vi "CBSControlling.vi"() -> ()   [LabVIEW 2017]
uses:
  classes/DataHandlerMYiTOPS.lvclass
panel:
  out "Steps":u64
  out "NewVal":u64
  in  "Monitoring":T1 {"Meter" scale=0.0..20.0}
  out "appended array":string[](array[string])
  out "element":string
  out "Control-Matrix-Overview 2":i32(listbox)=-1
  in  "Controlling":T2={"LED 1"=FALSE, "Stop Client App"=FALSE, "LED 2"=FALSE, "Drive Motor"=FALSE, "Direcion Moter"=FALSE, "Steps"=512} {"Steps" min=1 step=1}
  in  "Cyber-physical Objects":i32(listbox)
  in  "Stop":bool
  out "Control-Matrix-Overview":i32(listbox)=-1
  # "Hard Key:"
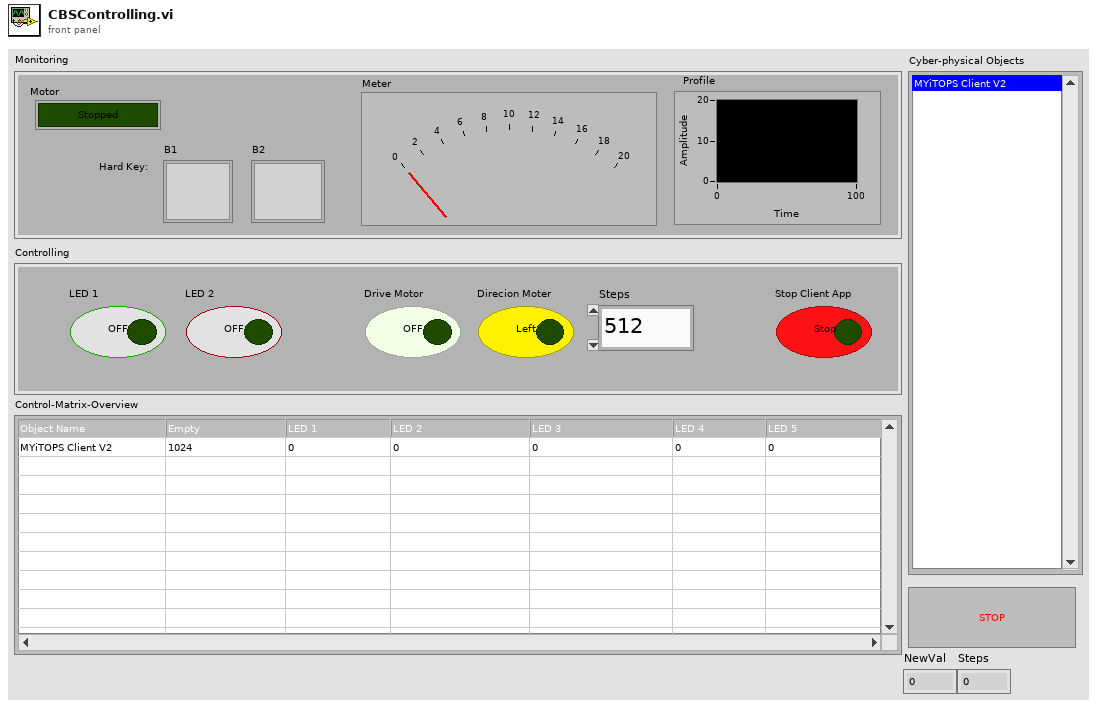
[diagram p1: front panel]
types:
  T1 = cluster{"Meter":i8, "Profile":dbl, "B2":bool, "B1":bool, "Motor":bool}
  T2 = cluster{"LED 1":bool, "Stop Client App":bool, "LED 2":bool, "Drive Motor":bool, "Direcion Moter":bool, "Steps":u64}
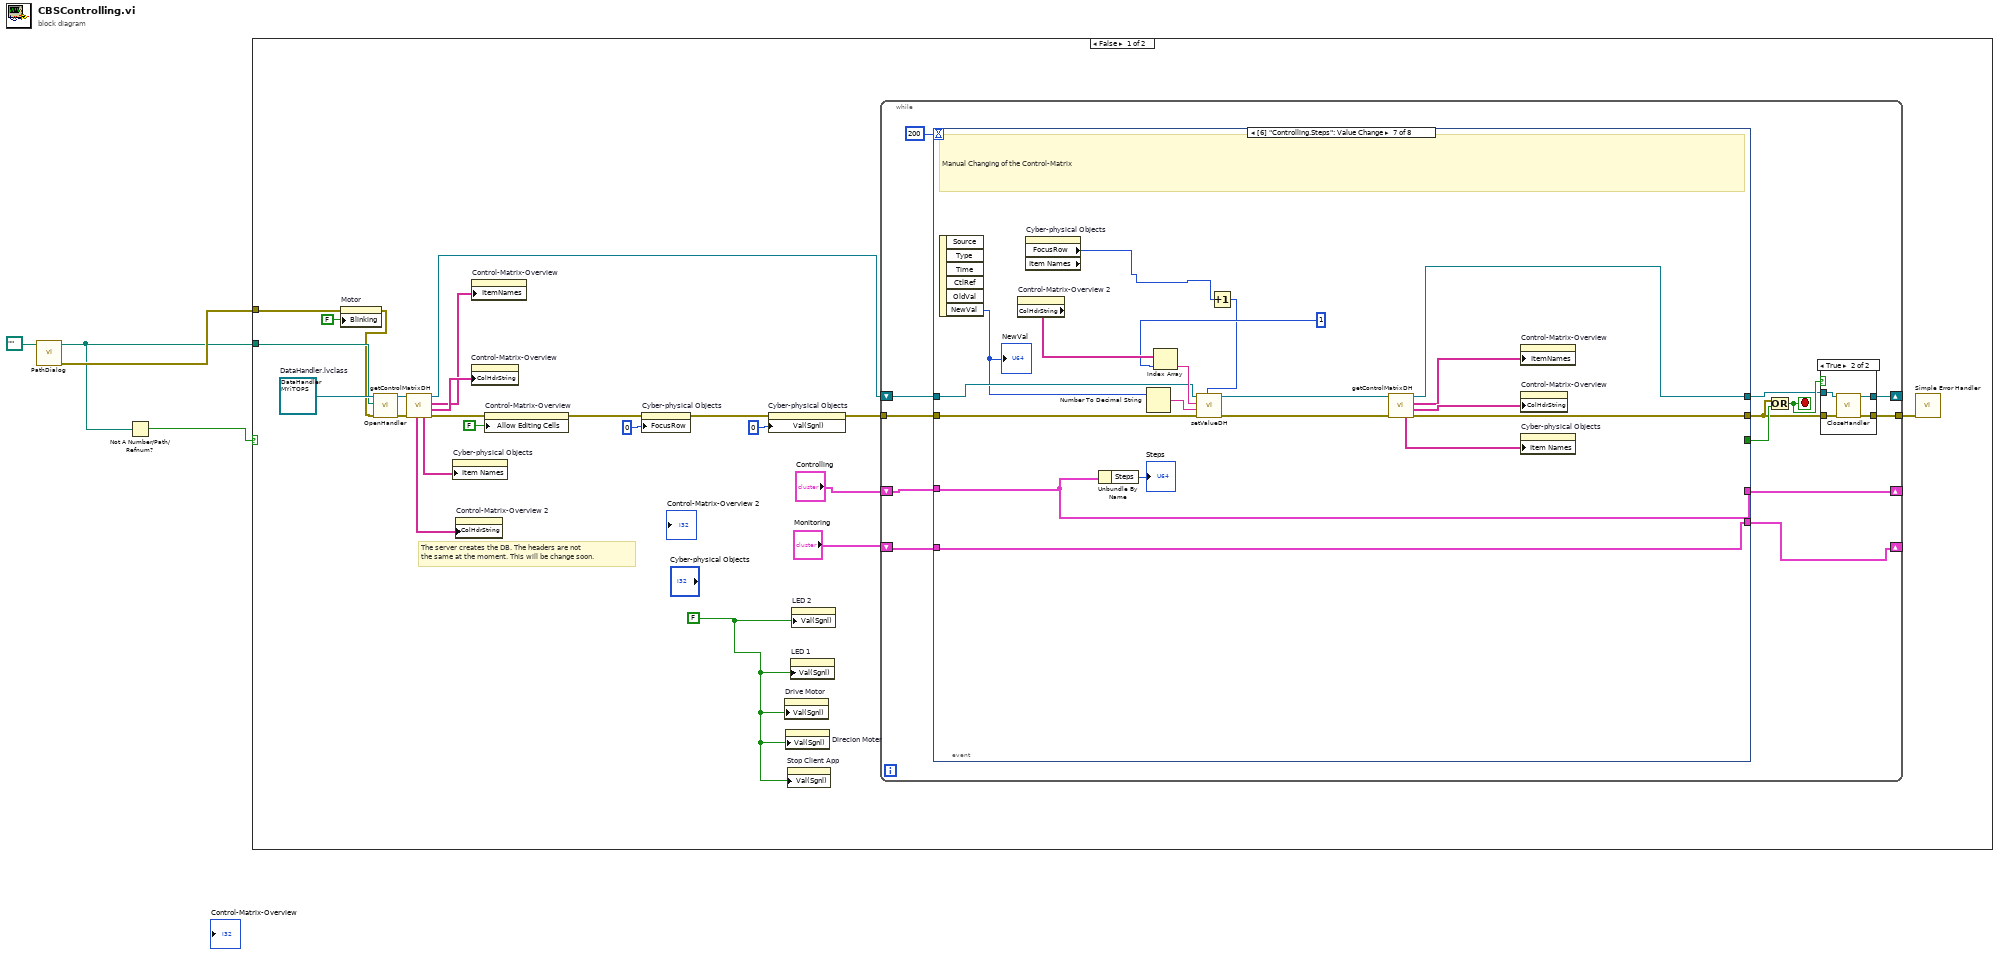
[diagram p0: block diagram]
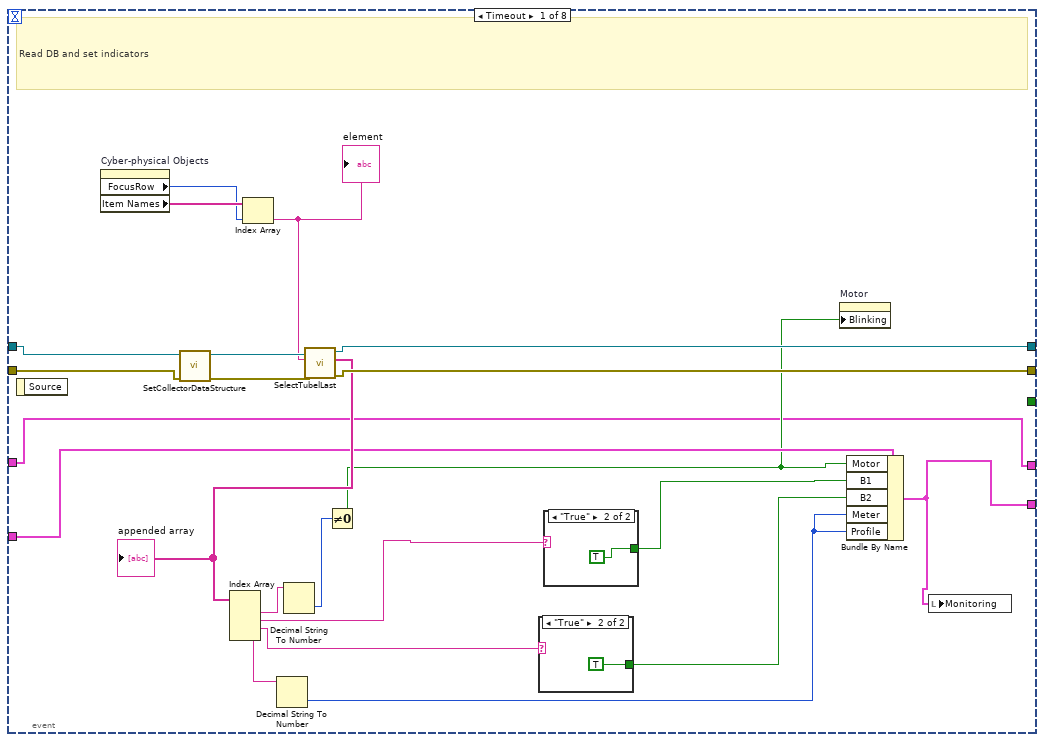
[diagram p3: hidden frame]
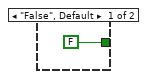
[diagram p4: hidden frame]
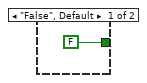
[diagram p5: hidden frame]
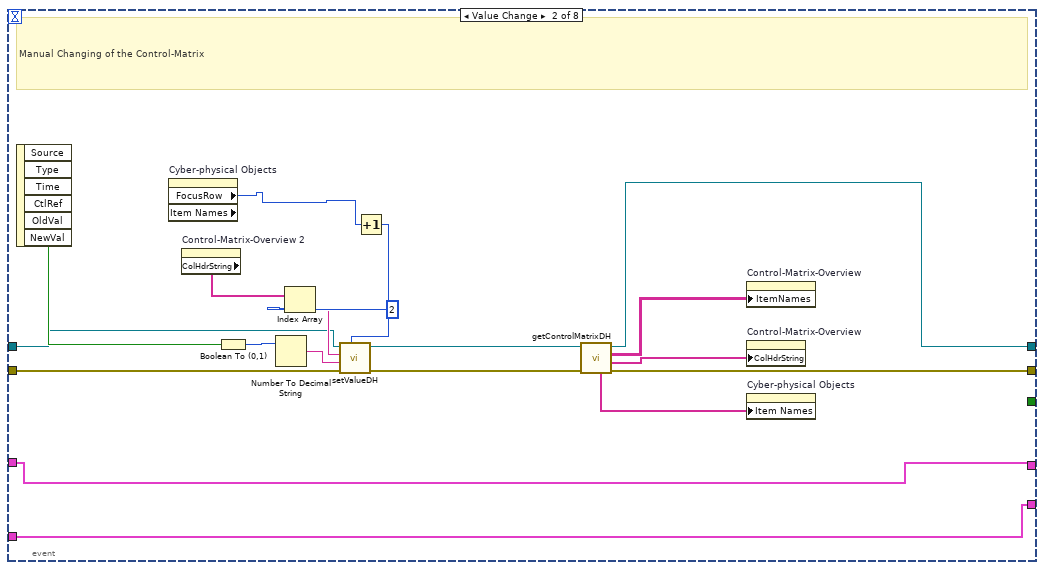
[diagram p6: hidden frame]
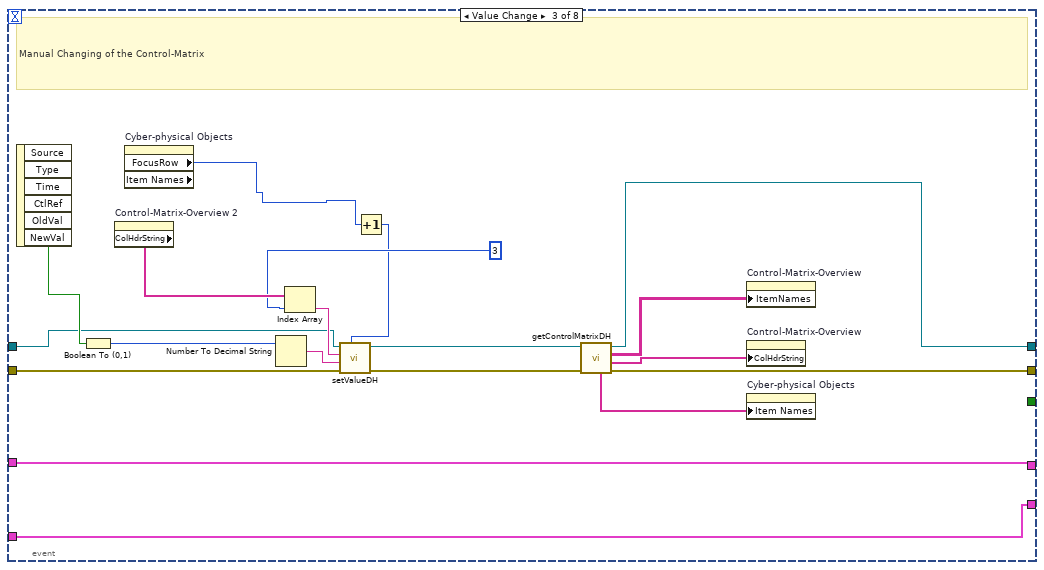
[diagram p7: hidden frame]
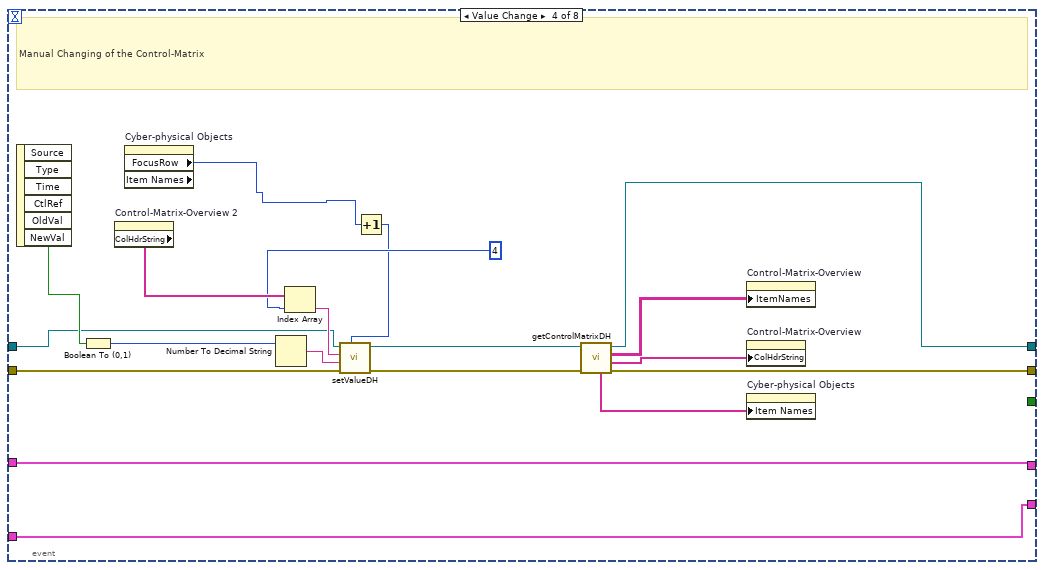
[diagram p8: hidden frame]
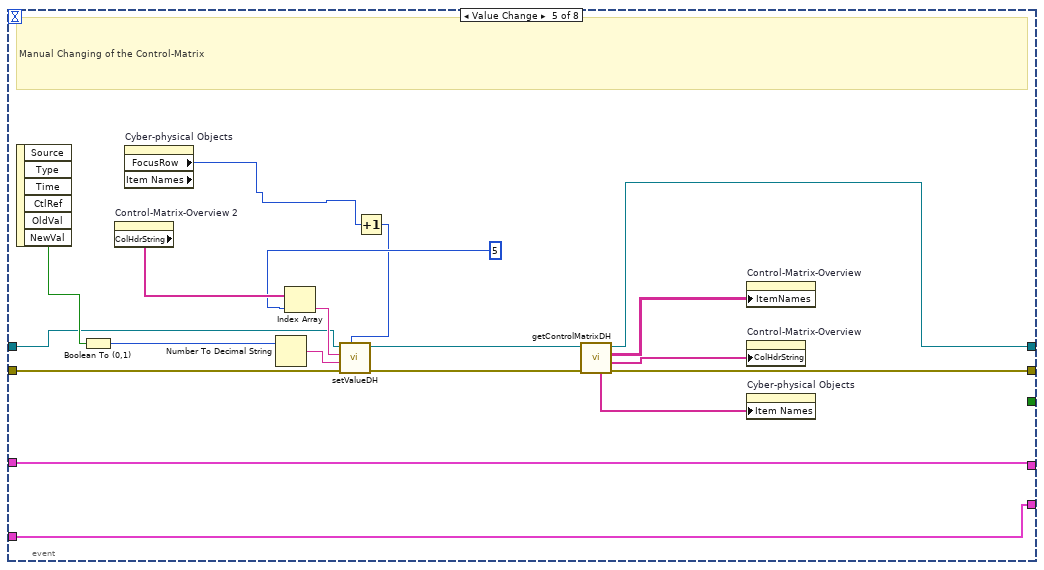
[diagram p9: hidden frame]
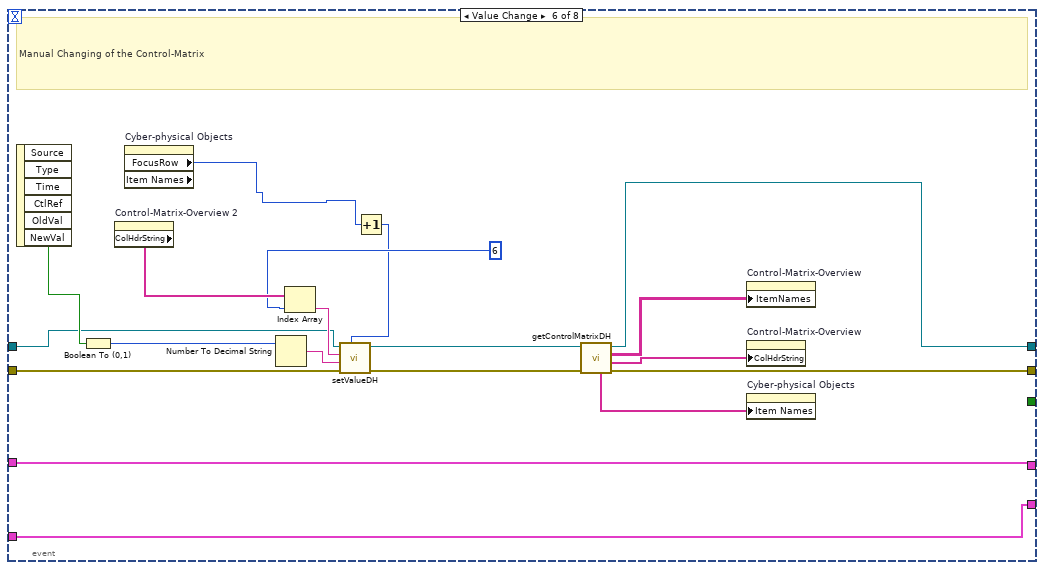
[diagram p10: hidden frame]
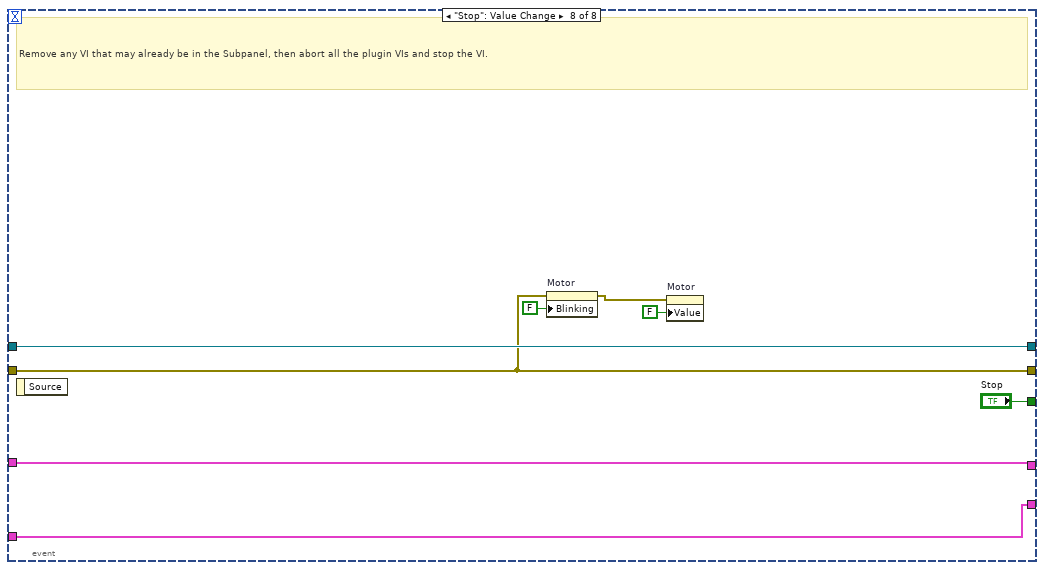
[diagram p11: hidden frame]
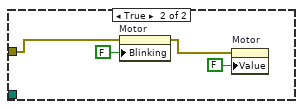
[diagram p12: hidden frame]
diagram:
  n1 = call "PathDialog.vi"("Path to Data Base in"=path "" ("Path to Data Base")) -> ("error out"=w3:errorcluster, "Path to Data Base out"=w2:path)  [unwired: 9 in]
  n2 = Not A Number/Path/Refnum?(number/path/refnum=w2) -> (NaN/Path/Refnum?=w1:bool)
  n3 = case shown="False" w1 {
    tunnel: w2 -> [w10 _]
    tunnel: w3 -> [w7 w197]
    frame False {
      w8 = FALSE ("Value")
      w23 = refnum<class "DataHandlerMYiTOPS.lvclass"> refnum  # DataHandler.lvclass
      # "The server creates the DB. The headers are not \nthe same at the moment. This will be change soon."
      n4 = property on="Motor" class="Bool (strict)"(error in=w7, "Blinking"=FALSE) -> (error out=w6:errorcluster)  [unwired: 1 in, 1 out]
      n5 = call-dynamic "OpenHandler.vi"("error in (no error)"=w6, "path to db monitoring"=w10, "DataHandling in"=w23) -> ("error out"=w22:errorcluster, "DataHandling out"=w21:refnum<class "DataHandlerMYiTOPS.lvclass">)  [unwired: 7 in]
      n6 = call-dynamic "getControlMatrixDH.vi"("error in (no error)"=w22, "DataHandler in"=w21) -> ("error out"=w19:errorcluster, "List of ColHads"=w18:string[], "Array"=w13:string[][], "DataHandler out"=w14:refnum<class "DataHandlerMYiTOPS.lvclass">, "Field Elements"=w20:string[], "List of ColHads 2"=w12:string[])  [unwired: 4 in]
      n7 = property on="Cyber-physical Objects" class="LstBox (strict)"("Item Names"=w20) -> ()  [unwired: 2 in, 2 out]
      n8 = property on="Control-Matrix-Overview 2" class="MCListbox (strict)"("ColHdrString"=w12) -> ()  [unwired: 2 in, 2 out]
      n9 = property on="Control-Matrix-Overview" class="MCListbox (strict)"("ColHdrString"=w18) -> ()  [unwired: 2 in, 2 out]
      n10 = property on="Control-Matrix-Overview" class="MCListbox (strict)"("ItemNames"=w13) -> ()  [unwired: 2 in, 2 out]
      n11 = property on="Control-Matrix-Overview" class="MCListbox (strict)"(error in=w19, "Allow Editing Cells"=FALSE) -> (error out=w15:errorcluster)  [unwired: 1 in, 1 out]
      n12 = property on="Cyber-physical Objects" class="LstBox (strict)"(error in=w15, "FocusRow"=0 ("Focus Row")) -> (error out=w16:errorcluster)  [unwired: 1 in, 1 out]
      n13 = property on="Cyber-physical Objects" class="ListBox (strict)"(error in=w16, "Val(Sgnl)"=u16 0 ("Value (Signaling)")) -> (error out=w27:errorcluster)  [unwired: 1 in, 1 out]
      n14 = property on="Drive Motor" class="Bool (strict)"("Val(Sgnl)"=w8) -> ()  [unwired: 2 in, 2 out]
      n15 = property on="Direcion Moter" class="Bool (strict)"("Val(Sgnl)"=w8) -> ()  [unwired: 2 in, 2 out]
      n16 = property on="Stop Client App" class="Bool (strict)"("Val(Sgnl)"=w8) -> ()  [unwired: 2 in, 2 out]
      n17 = property on="LED 1" class="Bool (strict)"("Val(Sgnl)"=w8) -> ()  [unwired: 2 in, 2 out]
      n18 = property on="LED 2" class="Bool (strict)"("Val(Sgnl)"=w8) -> ()  [unwired: 2 in, 2 out]
      n19 = while {
        tunnel: w27 -> [w39]
        tunnel: [w34] -> w25
        shift-right: [w32] -> _
        shift-left: w14 -> [w37]
        shift-right: [w28] -> _
        shift-left: "Controlling" -> [w31]
        shift-right: [w29] -> _
        shift-left: "Monitoring" -> [w30]
        stop <- w36 stop-if-true
        n20 = event shown="[6] \"Controlling.Steps\": Value Change" {
          selector: _ -> [_ _ _ _ _ _ _ _]
          dyn-events: _ -> [_ _ _ _ _ _ _ _]
          timeout: 200 -> [_ _ _ _ _ _ _ _]
          tunnel: [_ _ _ _ _ _ _ "Stop"] -> w40
          tunnel: [w61 w89 w106 w125 w144 w163 w182 w189] -> w35
          tunnel: w39 -> [w63 w91 w110 w129 w148 w167 w186 w189]
          tunnel: w37 -> [w66 w80 w97 w116 w135 w154 w175 w193]
          tunnel: [w64 w81 w98 w117 w136 w155 w176 w193] -> w33
          tunnel: w31 -> [w47 w77 w93 w112 w131 w150 w169 w192]
          tunnel: [w47 w77 w93 w112 w131 w150 w169 w192] -> w28
          tunnel: w30 -> [w51 w76 w92 w111 w130 w149 w171 w191]
          tunnel: [w50 w76 w92 w111 w130 w149 w171 w191] -> w29
          event Timeout {
            # "Read DB and set indicators"
            n21 = event-data() -> ()  [unwired: 1 in, 1 out]
            n22 = property on="Cyber-physical Objects" class="LstBox (strict)"() -> ("FocusRow"=w67:i32, "Item Names"=w68:string[])  [unwired: 2 in, 2 out]
            n23 = call-dynamic "SetCollectorDataStructure.vi"("error in (no error)"=w63, "DataHandler in"=w66) -> ("error out"=w62:errorcluster, "DataHandler out"=w65:refnum<class "DataHandlerMYiTOPS.lvclass">)  [unwired: 8 in]
            n24 = Index Array(array=w68, index=w67) -> (element=w60:string)
            "element" <- w60
            n25 = call-dynamic "SelectTubelLast.vi"("error in (no error)"=w62, "Unique Object Identifier"=w60, "DataHandler in"=w65) -> ("error out"=w61:errorcluster, "appended array"=w59:string[], "DataHandler out"=w64:refnum<class "DataHandlerMYiTOPS.lvclass">)  [unwired: 6 in]
            "appended array" <- w59
            n26 = Index Array(array=w59) -> (element #1=w58:string, element #2=w57:string, element #3=w56:string, element #4=w55:string)  [unwired: 4 in]
            n27 = Decimal String To Number(string=w55) -> (number=w54:i32)  [unwired: 2 in, 1 out]
            n28 = Decimal String To Number(string=w58) -> (number=w49:i32)  [unwired: 2 in, 1 out]
            n29 = Not Equal To 0?(x=w49) -> (x != 0?=w48:bool)
            n30 = case shown="\"True\"" w56 {
              tunnel: [FALSE TRUE] -> w53
              frame "False", Default {
              }
              frame "True" {
              }
            }
            n31 = case shown="\"True\"" w57 {
              tunnel: [FALSE TRUE] -> w52
              frame "False", Default {
              }
              frame "True" {
              }
            }
            n32 = property on="Motor" class="Bool (strict)"("Blinking"=w48) -> ()  [unwired: 2 in, 2 out]
            n33 = Bundle By Name(cluster=w51, "Motor"=w48, "B1"=w52, "B2"=w53, "Meter"=w54, "Profile"=w54) -> (w50:T1)
            n34 = local write "Monitoring"(w50) -> ()
          }
          event "Controlling.LED 1": Value Change {
            # "Manual Changing of the Control-Matrix"
            n35 = event-data() -> ("NewVal"=w84:bool)  [unwired: 1 in, 5 out]
            n36 = property on="Cyber-physical Objects" class="LstBox (strict)" props=["FocusRow", "Item Names"]() -> ("FocusRow"=w79:i32)  [unwired: 2 in, 3 out]
            n37 = property on="Control-Matrix-Overview 2" class="MCListbox (strict)"() -> ("ColHdrString"=w87:string[])  [unwired: 2 in, 2 out]
            n38 = Boolean To (0,1)(Boolean=w84) -> (0, 1=w83:i16)
            n39 = Number To Decimal String(number=w83) -> (decimal integer string=w88:string)  [unwired: 1 in]
            n40 = Index Array(array=w87, index=2) -> (element=w85:string)
            n41 = Increment(x=w79) -> (x+1=w78:i32)
            n42 = call-dynamic "setValueDH.vi"("Focus"=w78, "error in (no error)"=w91, "Value"=w88, "ItemName"=w85, "DataHandler in"=w80) -> ("error out"=w90:errorcluster, "DataHandler out"=w82:refnum<class "DataHandlerMYiTOPS.lvclass">)  [unwired: 5 in]
            n43 = call-dynamic "getControlMatrixDH.vi"("error in (no error)"=w90, "DataHandler in"=w82) -> ("error out"=w89:errorcluster, "List of ColHads"=w74:string[], "Array"=w73:string[][], "DataHandler out"=w81:refnum<class "DataHandlerMYiTOPS.lvclass">, "Field Elements"=w75:string[])  [unwired: 4 in, 1 out]
            n44 = property on="Control-Matrix-Overview" class="MCListbox (strict)"("ItemNames"=w73) -> ()  [unwired: 2 in, 2 out]
            n45 = property on="Control-Matrix-Overview" class="MCListbox (strict)"("ColHdrString"=w74) -> ()  [unwired: 2 in, 2 out]
            n46 = property on="Cyber-physical Objects" class="LstBox (strict)"("Item Names"=w75) -> ()  [unwired: 2 in, 2 out]
          }
          event "Controlling.LED 2": Value Change {
            # "Manual Changing of the Control-Matrix"
            n47 = event-data() -> ("NewVal"=w101:bool)  [unwired: 1 in, 5 out]
            n48 = Boolean To (0,1)(Boolean=w101) -> (0, 1=w100:i16)
            n49 = property on="Control-Matrix-Overview 2" class="MCListbox (strict)"() -> ("ColHdrString"=w104:string[])  [unwired: 2 in, 2 out]
            n50 = property on="Cyber-physical Objects" class="LstBox (strict)" props=["FocusRow", "Item Names"]() -> ("FocusRow"=w95:i32)  [unwired: 2 in, 3 out]
            n51 = Number To Decimal String(number=w100) -> (decimal integer string=w105:string)  [unwired: 1 in]
            n52 = Index Array(array=w104, index=3) -> (element=w102:string)
            n53 = Increment(x=w95) -> (x+1=w94:i32)
            n54 = call-dynamic "setValueDH.vi"("Focus"=w94, "error in (no error)"=w110, "Value"=w105, "ItemName"=w102, "DataHandler in"=w97) -> ("error out"=w107:errorcluster, "DataHandler out"=w99:refnum<class "DataHandlerMYiTOPS.lvclass">)  [unwired: 5 in]
            n55 = call-dynamic "getControlMatrixDH.vi"("error in (no error)"=w107, "DataHandler in"=w99) -> ("error out"=w106:errorcluster, "List of ColHads"=w108:string[], "Array"=w96:string[][], "DataHandler out"=w98:refnum<class "DataHandlerMYiTOPS.lvclass">, "Field Elements"=w109:string[])  [unwired: 4 in, 1 out]
            n56 = property on="Control-Matrix-Overview" class="MCListbox (strict)"("ItemNames"=w96) -> ()  [unwired: 2 in, 2 out]
            n57 = property on="Control-Matrix-Overview" class="MCListbox (strict)"("ColHdrString"=w108) -> ()  [unwired: 2 in, 2 out]
            n58 = property on="Cyber-physical Objects" class="LstBox (strict)"("Item Names"=w109) -> ()  [unwired: 2 in, 2 out]
          }
          event "Controlling.Drive Motor": Value Change {
            # "Manual Changing of the Control-Matrix"
            n59 = event-data() -> ("NewVal"=w120:bool)  [unwired: 1 in, 5 out]
            n60 = Boolean To (0,1)(Boolean=w120) -> (0, 1=w119:i16)
            n61 = property on="Control-Matrix-Overview 2" class="MCListbox (strict)"() -> ("ColHdrString"=w123:string[])  [unwired: 2 in, 2 out]
            n62 = property on="Cyber-physical Objects" class="LstBox (strict)" props=["FocusRow", "Item Names"]() -> ("FocusRow"=w114:i32)  [unwired: 2 in, 3 out]
            n63 = Number To Decimal String(number=w119) -> (decimal integer string=w124:string)  [unwired: 1 in]
            n64 = Index Array(array=w123, index=4) -> (element=w121:string)
            n65 = Increment(x=w114) -> (x+1=w113:i32)
            n66 = call-dynamic "setValueDH.vi"("Focus"=w113, "error in (no error)"=w129, "Value"=w124, "ItemName"=w121, "DataHandler in"=w116) -> ("error out"=w126:errorcluster, "DataHandler out"=w118:refnum<class "DataHandlerMYiTOPS.lvclass">)  [unwired: 5 in]
            n67 = call-dynamic "getControlMatrixDH.vi"("error in (no error)"=w126, "DataHandler in"=w118) -> ("error out"=w125:errorcluster, "List of ColHads"=w127:string[], "Array"=w115:string[][], "DataHandler out"=w117:refnum<class "DataHandlerMYiTOPS.lvclass">, "Field Elements"=w128:string[])  [unwired: 4 in, 1 out]
            n68 = property on="Control-Matrix-Overview" class="MCListbox (strict)"("ItemNames"=w115) -> ()  [unwired: 2 in, 2 out]
            n69 = property on="Control-Matrix-Overview" class="MCListbox (strict)"("ColHdrString"=w127) -> ()  [unwired: 2 in, 2 out]
            n70 = property on="Cyber-physical Objects" class="LstBox (strict)"("Item Names"=w128) -> ()  [unwired: 2 in, 2 out]
          }
          event "Controlling.Direcion Moter": Value Change {
            # "Manual Changing of the Control-Matrix"
            n71 = event-data() -> ("NewVal"=w139:bool)  [unwired: 1 in, 5 out]
            n72 = Boolean To (0,1)(Boolean=w139) -> (0, 1=w138:i16)
            n73 = property on="Control-Matrix-Overview 2" class="MCListbox (strict)"() -> ("ColHdrString"=w142:string[])  [unwired: 2 in, 2 out]
            n74 = property on="Cyber-physical Objects" class="LstBox (strict)" props=["FocusRow", "Item Names"]() -> ("FocusRow"=w133:i32)  [unwired: 2 in, 3 out]
            n75 = Number To Decimal String(number=w138) -> (decimal integer string=w143:string)  [unwired: 1 in]
            n76 = Index Array(array=w142, index=5) -> (element=w140:string)
            n77 = Increment(x=w133) -> (x+1=w132:i32)
            n78 = call-dynamic "setValueDH.vi"("Focus"=w132, "error in (no error)"=w148, "Value"=w143, "ItemName"=w140, "DataHandler in"=w135) -> ("error out"=w145:errorcluster, "DataHandler out"=w137:refnum<class "DataHandlerMYiTOPS.lvclass">)  [unwired: 5 in]
            n79 = call-dynamic "getControlMatrixDH.vi"("error in (no error)"=w145, "DataHandler in"=w137) -> ("error out"=w144:errorcluster, "List of ColHads"=w146:string[], "Array"=w134:string[][], "DataHandler out"=w136:refnum<class "DataHandlerMYiTOPS.lvclass">, "Field Elements"=w147:string[])  [unwired: 4 in, 1 out]
            n80 = property on="Control-Matrix-Overview" class="MCListbox (strict)"("ItemNames"=w134) -> ()  [unwired: 2 in, 2 out]
            n81 = property on="Control-Matrix-Overview" class="MCListbox (strict)"("ColHdrString"=w146) -> ()  [unwired: 2 in, 2 out]
            n82 = property on="Cyber-physical Objects" class="LstBox (strict)"("Item Names"=w147) -> ()  [unwired: 2 in, 2 out]
          }
          event "Controlling.Stop Client App": Value Change {
            # "Manual Changing of the Control-Matrix"
            n83 = event-data() -> ("NewVal"=w158:bool)  [unwired: 1 in, 5 out]
            n84 = Boolean To (0,1)(Boolean=w158) -> (0, 1=w157:i16)
            n85 = property on="Control-Matrix-Overview 2" class="MCListbox (strict)"() -> ("ColHdrString"=w161:string[])  [unwired: 2 in, 2 out]
            n86 = property on="Cyber-physical Objects" class="LstBox (strict)" props=["FocusRow", "Item Names"]() -> ("FocusRow"=w152:i32)  [unwired: 2 in, 3 out]
            n87 = Number To Decimal String(number=w157) -> (decimal integer string=w162:string)  [unwired: 1 in]
            n88 = Index Array(array=w161, index=6) -> (element=w159:string)
            n89 = Increment(x=w152) -> (x+1=w151:i32)
            n90 = call-dynamic "setValueDH.vi"("Focus"=w151, "error in (no error)"=w167, "Value"=w162, "ItemName"=w159, "DataHandler in"=w154) -> ("error out"=w164:errorcluster, "DataHandler out"=w156:refnum<class "DataHandlerMYiTOPS.lvclass">)  [unwired: 5 in]
            n91 = call-dynamic "getControlMatrixDH.vi"("error in (no error)"=w164, "DataHandler in"=w156) -> ("error out"=w163:errorcluster, "List of ColHads"=w165:string[], "Array"=w153:string[][], "DataHandler out"=w155:refnum<class "DataHandlerMYiTOPS.lvclass">, "Field Elements"=w166:string[])  [unwired: 4 in, 1 out]
            n92 = property on="Control-Matrix-Overview" class="MCListbox (strict)"("ItemNames"=w153) -> ()  [unwired: 2 in, 2 out]
            n93 = property on="Control-Matrix-Overview" class="MCListbox (strict)"("ColHdrString"=w165) -> ()  [unwired: 2 in, 2 out]
            n94 = property on="Cyber-physical Objects" class="LstBox (strict)"("Item Names"=w166) -> ()  [unwired: 2 in, 2 out]
          }
          event "Controlling.Steps": Value Change {
            # "Manual Changing of the Control-Matrix"
            n95 = event-data() -> ("NewVal"=w170:u64)  [unwired: 1 in, 5 out]
            "NewVal" <- w170
            n96 = property on="Control-Matrix-Overview 2" class="MCListbox (strict)"() -> ("ColHdrString"=w180:string[])  [unwired: 2 in, 2 out]
            n97 = property on="Cyber-physical Objects" class="LstBox (strict)" props=["FocusRow", "Item Names"]() -> ("FocusRow"=w173:i32)  [unwired: 2 in, 3 out]
            n98 = Unbundle By Name(w169) -> ("Steps"=→"Steps":u64)
            n99 = Number To Decimal String(number=w170) -> (decimal integer string=w181:string)  [unwired: 1 in]
            n100 = Index Array(array=w180, index=1) -> (element=w178:string)
            n101 = Increment(x=w173) -> (x+1=w172:i32)
            n102 = call-dynamic "setValueDH.vi"("Focus"=w172, "error in (no error)"=w186, "Value"=w181, "ItemName"=w178, "DataHandler in"=w175) -> ("error out"=w183:errorcluster, "DataHandler out"=w177:refnum<class "DataHandlerMYiTOPS.lvclass">)  [unwired: 5 in]
            n103 = call-dynamic "getControlMatrixDH.vi"("error in (no error)"=w183, "DataHandler in"=w177) -> ("error out"=w182:errorcluster, "List of ColHads"=w184:string[], "Array"=w174:string[][], "DataHandler out"=w176:refnum<class "DataHandlerMYiTOPS.lvclass">, "Field Elements"=w185:string[])  [unwired: 4 in, 1 out]
            n104 = property on="Control-Matrix-Overview" class="MCListbox (strict)"("ItemNames"=w174) -> ()  [unwired: 2 in, 2 out]
            n105 = property on="Control-Matrix-Overview" class="MCListbox (strict)"("ColHdrString"=w184) -> ()  [unwired: 2 in, 2 out]
            n106 = property on="Cyber-physical Objects" class="LstBox (strict)"("Item Names"=w185) -> ()  [unwired: 2 in, 2 out]
          }
          event "Stop": Value Change {
            # "Remove any VI that may already be in the Subpanel, then abort all the plugin VIs and stop the VI."
            n107 = event-data() -> ()  [unwired: 1 in, 1 out]
            n108 = property on="Motor" class="Bool (strict)"(error in=w189, "Blinking"=FALSE) -> (error out=w188:errorcluster)  [unwired: 1 in, 1 out]
            n109 = property on="Motor" class="Bool (strict)"(error in=w188, "Value"=FALSE) -> ()  [unwired: 1 in, 2 out]
          }
        }
        n110 = Or(x=w35, y=w40) -> (x .or. y?=w36:bool)
        n111 = case shown="True" w36 {
          tunnel: w35 -> [w42 w45]
          tunnel: [w42 w46] -> w34
          tunnel: w33 -> [w41 w44]
          tunnel: [w41 w43] -> w32
          frame False {
          }
          frame True {
            n112 = call-dynamic "CloseHandler.vi"("error in (no error)"=w45, "DataHandling in"=w44) -> ("error out"=w46:errorcluster, "DataHandling out"=w43:refnum<class "DataHandlerMYiTOPS.lvclass">)  [unwired: 8 in]
          }
        }
      }
      n113 = call <vilib>:"Simple Error Handler.vi"("error in (no error)"=w25) -> ()  [unwired: 4 in, 5 out]
    }
    frame True {
      n114 = property on="Motor" class="Bool (strict)"(error in=w197, "Blinking"=FALSE) -> (error out=w195:errorcluster)  [unwired: 1 in, 1 out]
      n115 = property on="Motor" class="Bool (strict)"(error in=w195, "Value"=FALSE) -> ()  [unwired: 1 in, 2 out]
    }
  }
